vi "Read_Logger.vi"(4 "Input String":string, 5 "Msg In":u8=255, 6 "aDATA":u8[](array[numeric])) -> (0 "Output String":string, 1 "End of Log":bool, 2 "Msg out":u8=255, 3 "Send_Msg":bool)   [LabVIEW 2017]
panel:
  in  "Type of message":bool
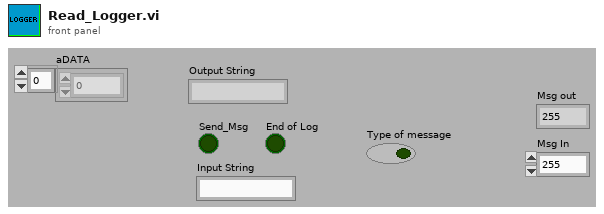
[diagram p1: front panel]
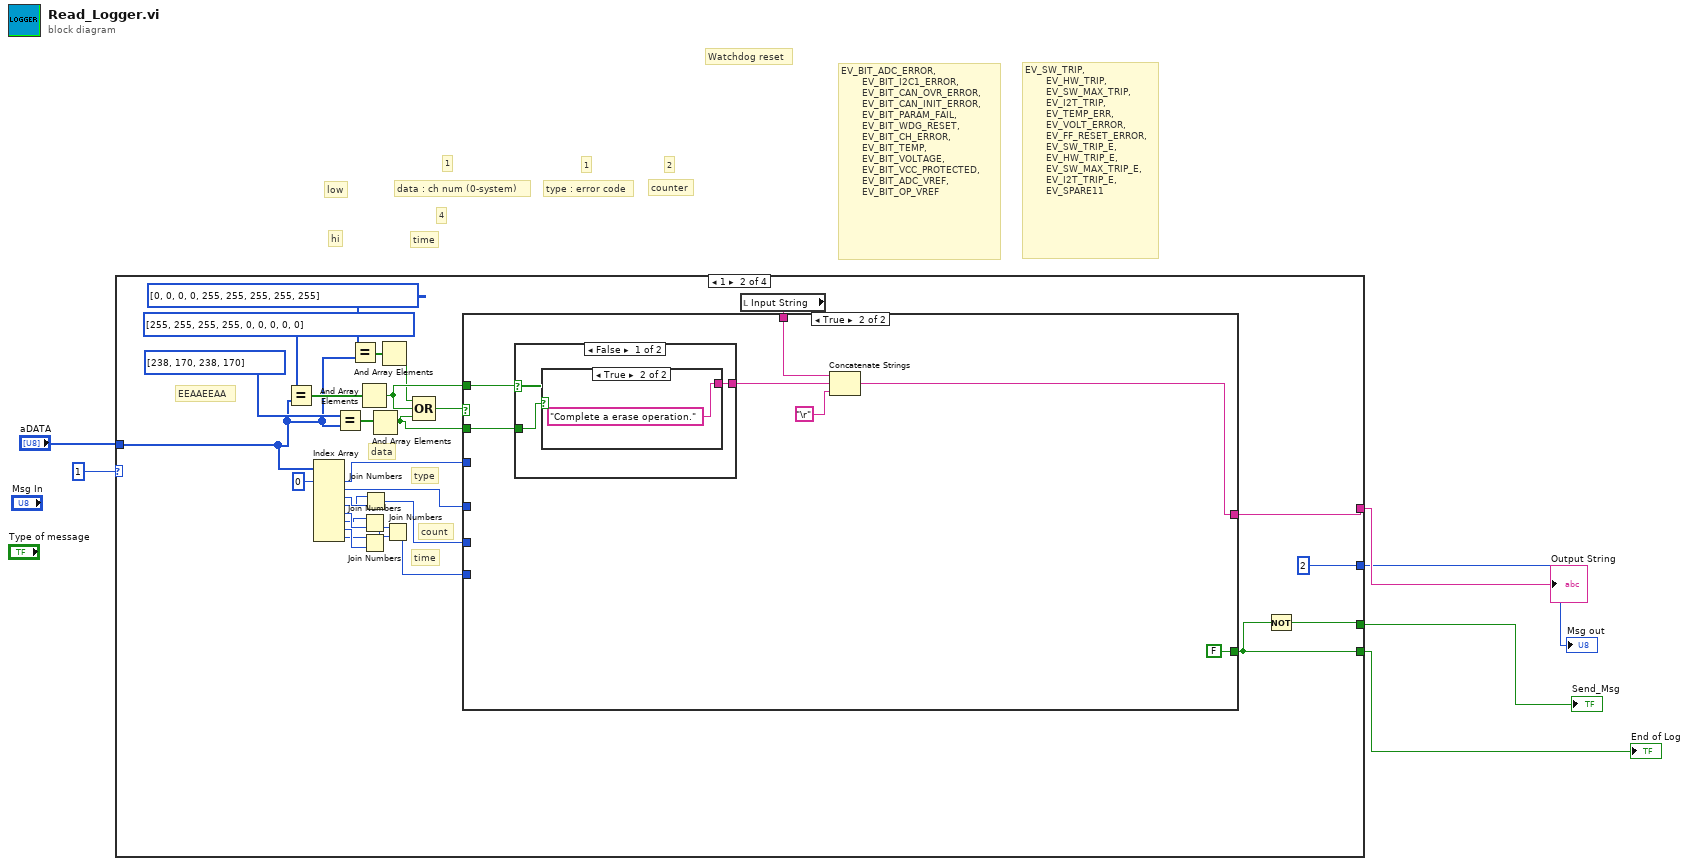
[diagram p0: block diagram]
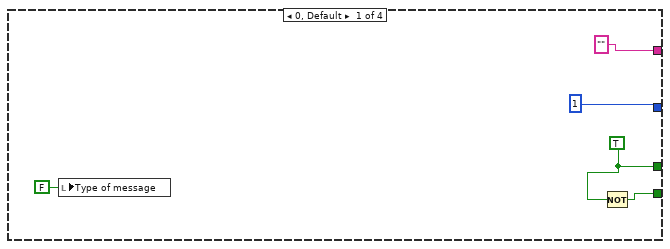
[diagram p2: hidden frame]
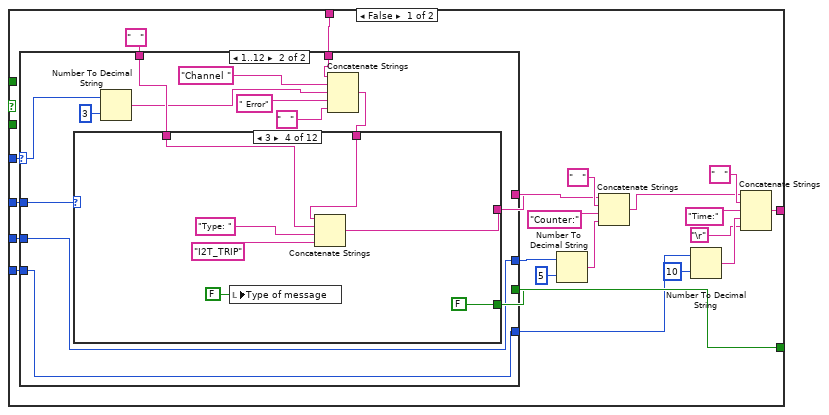
[diagram p3: hidden frame]
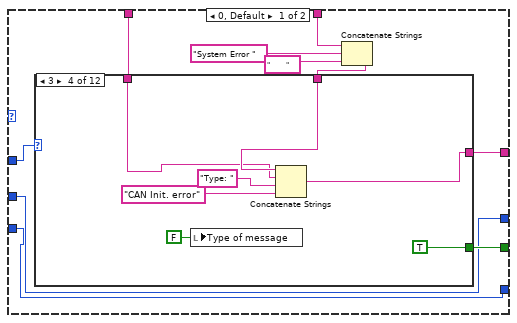
[diagram p4: hidden frame]
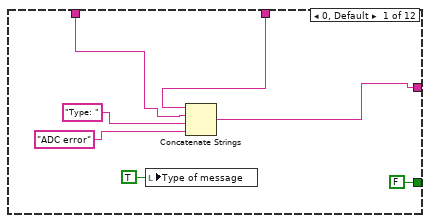
[diagram p5: hidden frame]
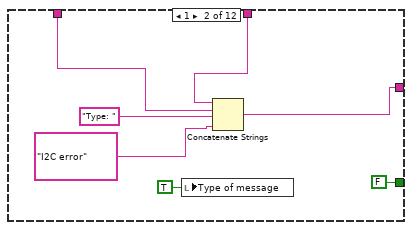
[diagram p6: hidden frame]
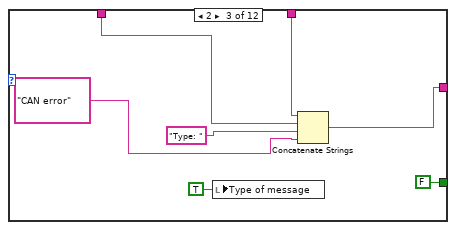
[diagram p7: hidden frame]
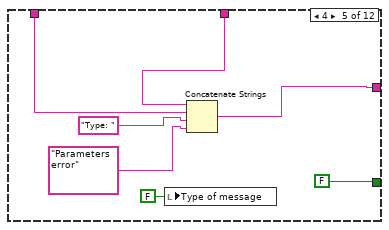
[diagram p8: hidden frame]
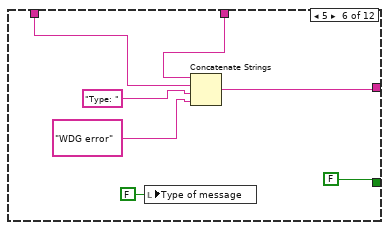
[diagram p9: hidden frame]
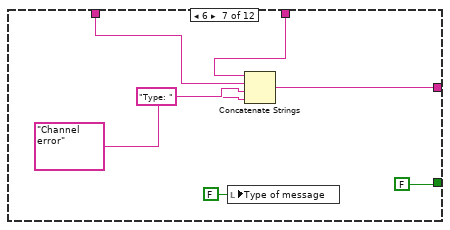
[diagram p10: hidden frame]
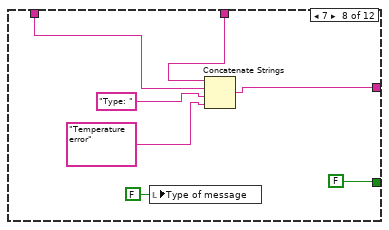
[diagram p11: hidden frame]
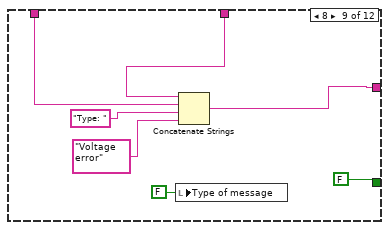
[diagram p12: hidden frame]
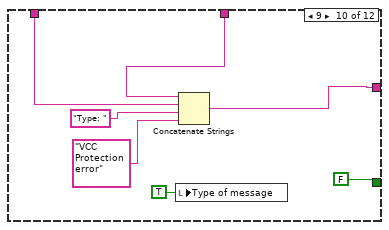
[diagram p13: hidden frame]
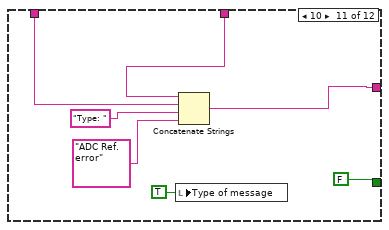
[diagram p14: hidden frame]
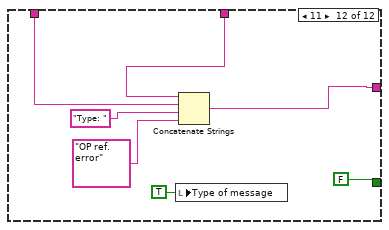
[diagram p15: hidden frame]
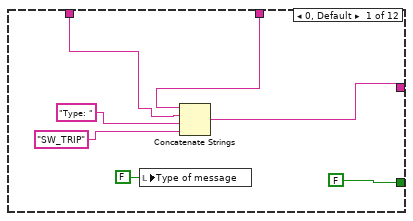
[diagram p16: hidden frame]
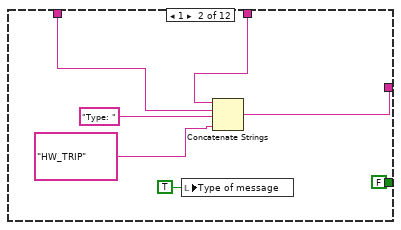
[diagram p17: hidden frame]
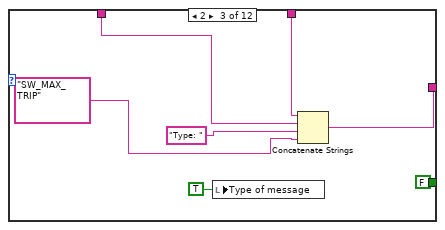
[diagram p18: hidden frame]
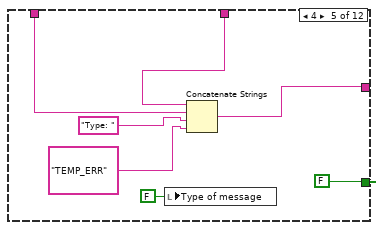
[diagram p19: hidden frame]
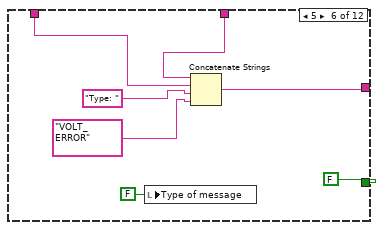
[diagram p20: hidden frame]
diagram:
  # "Watchdog reset"
  # "EV_SW_TRIP,\n       EV_HW_TRIP,\n       EV_SW_MAX_TRIP,\n       EV_I2T_TRIP,\n       EV_TEMP_ERR,\n       EV_VOLT_ERROR,\n       EV_FF_RESET_ERROR,\n       EV_SW_TRIP_E,\n       EV_HW_TRIP_E,\n       EV_SW_MAX_TRIP_E,\n       EV_I2T_TRIP_E,\n       EV_SPARE11"
  # "EV_BIT_ADC_ERROR,\n       EV_BIT_I2C1_ERROR,\n       EV_BIT_CAN_OVR_ERROR,\n       EV_BIT_CAN_INIT_ERROR,\n       EV_BIT_PARAM_FAIL,\n       EV_BIT_WDG_RESET,\n       EV_BIT_CH_ERROR,\n       EV_BIT_TEMP,\n       EV_BIT_VOLTAGE,\n       EV_BIT_VCC_PROTECTED,\n       EV_BIT_ADC_VREF,\n       EV_BIT_OP_VREF"
  # "4"
  # "time"
  # "hi"
  # "low"
  # "2"
  # "counter"
  # "1"
  # "1"
  # "type : error code"
  # "data : ch num (0-system)"
  n1 = case shown="1" u8 1 ("y") {
    tunnel: "aDATA" -> [_ w16 w292 _]
    tunnel: ["" w24 w282 "EEPROM has been erased."] -> w5
    tunnel: [u8 1 ("Type of msg in 2") u8 2 ("Type of msg in 2") u8 1 ("Type of msg in 2") u8 0 ("Type of msg in 2")] -> w4
    tunnel: [w8 w36 w268 FALSE ("Read_Log")] -> w3
    tunnel: [w9 w37 w267 FALSE ("End of log")] -> w2
    frame 0, Default {
      w8 = TRUE ("End of log")
      n2 = local write "Type of message"(FALSE ("Type of message")) -> ()
      n3 = Not(x=w8) -> (.not. x?=w9:bool)
    }
    frame 1 {
      # "EEAAEEAA"
      # "time"
      # "count"
      # "type"
      # "data"
      n4 = Equal?(x=u8[] [255, 255, 255, 255, 0, 0, 0, 0, 0] ("aDATA"), y=w16) -> (x = y?=w21:bool[])
      n5 = Index Array(array=w16, index #1=0 ("index")) -> (element #1=w23:u8, element #2=w35:u8, element #3=w34:u8, element #4=w33:u8, element #5=w31:u8, element #6=w30:u8, element #7=w29:u8, element #8=w28:u8)  [unwired: 7 in]
      n6 = Equal?(x=u8[] [238, 170, 238, 170] ("aDATA"), y=w16) -> (x = y?=w19:bool[])
      n7 = Equal?(x=u8[] [0, 0, 0, 0, 255, 255, 255, 255, 255] ("aDATA"), y=w16) -> (x = y?=w15:bool[])
      n8 = And Array Elements(Boolean array=w21) -> (logical AND=w18:bool)
      n9 = Join Numbers(hi=w30, lo=w31) -> ((hi.lo)=w27:u16)
      n10 = Join Numbers(hi=w28, lo=w29) -> ((hi.lo)=w26:u16)
      n11 = Join Numbers(hi=w33, lo=w34) -> ((hi.lo)=w32:u16)
      n12 = And Array Elements(Boolean array=w19) -> (logical AND=w12:bool)
      n13 = And Array Elements(Boolean array=w15) -> (logical AND=w13:bool)
      n14 = Join Numbers(hi=w26, lo=w27) -> ((hi.lo)=w25:u32)
      n15 = Compound Arithmetic op=OR(w13, w18, w12) -> (w14:bool)
      n16 = local read "Input String"() -> (w38:string)
      n17 = case shown="True" w14 {
        tunnel: w38 -> [w61 w260]
        tunnel: [w60 FALSE ("Read_Log")] -> w37
        tunnel: w35 -> [w59 _]
        tunnel: w32 -> [w58 _]
        tunnel: w25 -> [w57 _]
        tunnel: [w43 w259] -> w24
        tunnel: w23 -> [w41 _]
        tunnel: w18 -> [_ w256]
        tunnel: w12 -> [_ w254]
        frame False {
          n18 = case shown="1..12" w41 {
            selector: w41 -> [_ w162]
            tunnel: [w64 w169] -> w52
            tunnel: w61 -> [w69 w165]
            tunnel: "   " -> [w71 w167]
            tunnel: [w70 w168] -> w60
            tunnel: w59 -> [w66 w159]
            tunnel: w58 -> [w63 w158]
            tunnel: w57 -> [w62 w157]
            tunnel: [w63 w158] -> w51
            tunnel: [w62 w157] -> w45
            frame 0, Default {
              n19 = Concatenate Strings(w69, "System Error " ("string"), "        ") -> (w67:string)
              n20 = case shown="3" w66 {
                tunnel: [w75 w84 w90 w99 w103 w110 w117 w124 w131 w138 w145 w152] -> w64
                tunnel: w67 -> [w76 w83 w89 w97 w106 w111 w118 w125 w128 w135 w142 w149]
                tunnel: w71 -> [w72 w79 w86 w96 w100 w107 w114 w121 w134 w141 w148 w155]
                tunnel: [FALSE ("Read_Log") FALSE ("Read_Log") FALSE ("Read_Log") TRUE ("Read_Log") FALSE ("Read_Log") FALSE ("Read_Log") FALSE ("Read_Log") FALSE ("Read_Log") FALSE ("Read_Log") FALSE ("Read_Log") FALSE ("Read_Log") FALSE ("Read_Log")] -> w70
                frame 0, Default {
                  n21 = local write "Type of message"(TRUE ("Type of message")) -> ()
                  n22 = Concatenate Strings(w76, w72, "Type: " ("string"), "ADC error" ("string")) -> (w75:string)
                }
                frame 1 {
                  n23 = local write "Type of message"(TRUE ("Type of message")) -> ()
                  n24 = Concatenate Strings(w83, w79, "Type: " ("string"), "I2C error" ("string")) -> (w84:string)
                }
                frame 2 {
                  n25 = local write "Type of message"(TRUE ("Type of message")) -> ()
                  n26 = Concatenate Strings(w89, w86, "Type: " ("string"), "CAN error" ("string")) -> (w90:string)
                }
                frame 3 {
                  n27 = local write "Type of message"(FALSE ("Type of message")) -> ()
                  n28 = Concatenate Strings(w97, w96, "Type: " ("string"), "CAN Init. error" ("string")) -> (w99:string)
                }
                frame 4 {
                  n29 = local write "Type of message"(FALSE ("Type of message")) -> ()
                  n30 = Concatenate Strings(w106, w100, "Type: " ("string"), "Parameters error" ("string")) -> (w103:string)
                }
                frame 5 {
                  n31 = local write "Type of message"(FALSE ("Type of message")) -> ()
                  n32 = Concatenate Strings(w111, w107, "Type: " ("string"), "WDG error" ("string")) -> (w110:string)
                }
                frame 6 {
                  n33 = local write "Type of message"(FALSE ("Type of message")) -> ()
                  n34 = Concatenate Strings(w118, w114, "Type: " ("string"), "Channel error" ("string")) -> (w117:string)
                }
                frame 7 {
                  n35 = local write "Type of message"(FALSE ("Type of message")) -> ()
                  n36 = Concatenate Strings(w125, w121, "Type: " ("string"), "Temperature error" ("string")) -> (w124:string)
                }
                frame 8 {
                  n37 = local write "Type of message"(FALSE ("Type of message")) -> ()
                  n38 = Concatenate Strings(w128, w134, "Type: " ("string"), "Voltage error" ("string")) -> (w131:string)
                }
                frame 9 {
                  n39 = local write "Type of message"(TRUE ("Type of message")) -> ()
                  n40 = Concatenate Strings(w135, w141, "Type: " ("string"), "VCC Protection error" ("string")) -> (w138:string)
                }
                frame 10 {
                  n41 = local write "Type of message"(TRUE ("Type of message")) -> ()
                  n42 = Concatenate Strings(w142, w148, "Type: " ("string"), "ADC Ref. error" ("string")) -> (w145:string)
                }
                frame 11 {
                  n43 = local write "Type of message"(TRUE ("Type of message")) -> ()
                  n44 = Concatenate Strings(w149, w155, "Type: " ("string"), "OP ref. error" ("string")) -> (w152:string)
                }
              }
            }
            frame 1..12 {
              n45 = Number To Decimal String(number=w162, width (-)=i16 3) -> (decimal integer string=w160:string)
              n46 = Concatenate Strings(w165, "Channel " ("string"), w160, " Error" ("string"), "   ") -> (w163:string)
              n47 = case shown="3" w159 {
                tunnel: [w173 w182 w188 w197 w201 w208 w215 w222 w229 w236 w243 w250] -> w169
                tunnel: w163 -> [w174 w181 w187 w192 w204 w209 w216 w223 w226 w233 w240 w247]
                tunnel: w167 -> [w170 w177 w184 w191 w198 w205 w212 w219 w232 w239 w246 w253]
                tunnel: [FALSE ("Read_Log") FALSE ("Read_Log") FALSE ("Read_Log") FALSE ("Read_Log") FALSE ("Read_Log") FALSE ("Read_Log") FALSE ("Read_Log") FALSE ("Read_Log") FALSE ("Read_Log") FALSE ("Read_Log") FALSE ("Read_Log") FALSE ("Read_Log")] -> w168
                frame 0, Default {
                  n48 = local write "Type of message"(FALSE ("Type of message")) -> ()
                  n49 = Concatenate Strings(w174, w170, "Type: " ("string"), "SW_TRIP" ("string")) -> (w173:string)
                }
                frame 1 {
                  n50 = local write "Type of message"(TRUE ("Type of message")) -> ()
                  n51 = Concatenate Strings(w181, w177, "Type: " ("string"), "HW_TRIP" ("string")) -> (w182:string)
                }
                frame 2 {
                  n52 = local write "Type of message"(TRUE ("Type of message")) -> ()
                  n53 = Concatenate Strings(w187, w184, "Type: " ("string"), "SW_MAX_TRIP" ("string")) -> (w188:string)
                }
                frame 3 {
                  n54 = local write "Type of message"(FALSE ("Type of message")) -> ()
                  n55 = Concatenate Strings(w192, w191, "Type: " ("string"), "I2T_TRIP" ("string")) -> (w197:string)
                }
                frame 4 {
                  n56 = local write "Type of message"(FALSE ("Type of message")) -> ()
                  n57 = Concatenate Strings(w204, w198, "Type: " ("string"), "TEMP_ERR" ("string")) -> (w201:string)
                }
                frame 5 {
                  n58 = local write "Type of message"(FALSE ("Type of message")) -> ()
                  n59 = Concatenate Strings(w209, w205, "Type: " ("string"), "VOLT_ERROR" ("string")) -> (w208:string)
                }
                frame 6 {
                  n60 = local write "Type of message"(FALSE ("Type of message")) -> ()
                  n61 = Concatenate Strings(w216, w212, "Type: " ("string"), "FF_RESET_ERROR" ("string")) -> (w215:string)
                }
                frame 7 {
                  n62 = local write "Type of message"(FALSE ("Type of message")) -> ()
                  n63 = Concatenate Strings(w223, w219, "Type: " ("string"), "SW_TRIP_E" ("string")) -> (w222:string)
                }
                frame 8 {
                  n64 = local write "Type of message"(FALSE ("Type of message")) -> ()
                  n65 = Concatenate Strings(w226, w232, "Type: " ("string"), "HW_TRIP_E" ("string")) -> (w229:string)
                }
                frame 9 {
                  n66 = local write "Type of message"(TRUE ("Type of message")) -> ()
                  n67 = Concatenate Strings(w233, w239, "Type: " ("string"), "SW_MAX_TRIP_E" ("string")) -> (w236:string)
                }
                frame 10 {
                  n68 = local write "Type of message"(TRUE ("Type of message")) -> ()
                  n69 = Concatenate Strings(w240, w246, "Type: " ("string"), "I2T_TRIP_E" ("string")) -> (w243:string)
                }
                frame 11 {
                  n70 = local write "Type of message"(TRUE ("Type of message")) -> ()
                  n71 = Concatenate Strings(w247, w253, "Type: " ("string"), "SPARE11" ("string")) -> (w250:string)
                }
              }
            }
          }
          n72 = Number To Decimal String(number=w51, width (-)=i16 5) -> (decimal integer string=w50:string)
          n73 = Concatenate Strings(w52, "   ", "Counter:" ("string"), w50) -> (w47:string)
          n74 = Number To Decimal String(number=w45, width (-)=i16 10) -> (decimal integer string=w44:string)
          n75 = Concatenate Strings(w47, "   ", "Time:" ("string"), w44, "\r") -> (w43:string)
        }
        frame True {
          n76 = case shown="False" w256 {
            tunnel: [w262 "Please close all channels." ("string")] -> w258
            tunnel: w254 -> [w261 _]
            frame False {
              n77 = case shown="True" w261 {
                tunnel: ["Logger Error !!!" ("string") "Complete a erase operation." ("string")] -> w262
                frame False {
                }
                frame True {
                }
              }
            }
            frame True {
            }
          }
          n78 = Concatenate Strings(w260, w258, "\r") -> (w259:string)
        }
      }
      n79 = Not(x=w37) -> (.not. x?=w36:bool)
    }
    frame 2 {
      n80 = Index Array(array=w292, index #1=0 ("index")) -> (element #1=w277:u8, element #2=w278:u8, element #3=w276:u8, element #4=w275:u8, element #5=w272:u8, element #6=w271:u8, element #7=w274:u8, element #8=w273:u8)  [unwired: 7 in]
      n81 = Join Numbers(hi=w278, lo=w277) -> ((hi.lo)=w289:u16)
      n82 = Join Numbers(hi=w275, lo=w276) -> ((hi.lo)=w290:u16)
      n83 = Join Numbers(hi=w271, lo=w272) -> ((hi.lo)=w287:u16)
      n84 = Join Numbers(hi=w273, lo=w274) -> ((hi.lo)=w286:u16)
      n85 = Join Numbers(hi=w290, lo=w289) -> ((hi.lo)=w280:u32)
      n86 = Join Numbers(hi=w286, lo=w287) -> ((hi.lo)=w270:u32)
      n87 = Increment(x=w270) -> (x+1=w269:u32)
      n88 = Number To Decimal String(number=w280) -> (decimal integer string=w288:string)  [unwired: 1 in]
      n89 = Number To Decimal String(number=w269) -> (decimal integer string=w285:string)  [unwired: 1 in]
      n90 = Not Equal?(x=w280, y=u32 4294967295) -> (x != y?=w268:bool)
      n91 = local read "Type of message"() -> (w266:bool)
      n92 = Not(x=w268) -> (.not. x?=w267:bool)
      n93 = case shown="False" w266 {
        tunnel: w288 -> [w294 w305]
        tunnel: w285 -> [_ w303]
        tunnel: "Input String" -> [w298 w302]
        tunnel: "\r" -> [w297 w301]
        tunnel: [w296 w300] -> w282
        frame False {
          n94 = Concatenate Strings(w298, w297, "Time Stamp: " ("string"), w294, "\r") -> (w296:string)
        }
        frame True {
          n95 = Concatenate Strings(w302, w301, "Time Stamp: " ("string"), w305, " Channel: " ("string"), w303, "\r") -> (w300:string)
        }
      }
    }
    frame 3 {
    }
  }
  "Output String" <- w5
  "Msg out" <- w4
  "Send_Msg" <- w3
  "End of Log" <- w2
